vi "Test Refresh Active Path is First.vi"(8 "error in (no error)":errorcluster) -> (0 "error out":errorcluster)   [LabVIEW 2019]
uses:
  Setting Database/Setting Database.lvclass
  C:/Program Files (x86)/National Instruments/LabVIEW 2019/vi.lib/JKI/JKI SMO/SMO/SMO.lvclass
  ObjectSettings/ObjectSettings.lvclass/ObjectSettings.ctl
  ObjectSettings/Accessors/Read Enabled.vi
  ObjectSettings/Accessors/Write Enabled.vi
  Path Settings/Path Settings.lvclass
  C:/Users/Albro/Documents/GitHub/AFM-Lithography/lvsrc/Classes/Settings/ObjectSettings/ObjectSettings.lvclass
  <vilib>/addons/_JKI Toolkits/Caraya/classes/Assert/Assert Equal Value_Variant.vi
  <vilib>/addons/_JKI Toolkits/Caraya/classes/Test/Test.lvclass
  <vilib>/addons/_JKI Toolkits/Caraya/classes/Assert/Assert.lvclass
  <vilib>/JKI/JKI SMO/SMO/SMO.lvclass
  <vilib>/LabVIEW Open Source Project/Unicity/RandomStringGenerator/RandomStringGenerator.lvclass
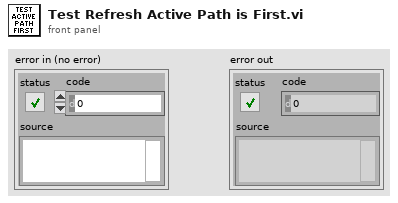
[diagram p1: front panel]
types:
  T1 = typedef "Setting Database.lvclass/PublicEvents--Cluster.ctl" = cluster{"NewActivePath":refnum<user-event>, "PathsUpdated":refnum<user-event>, "RectanglesUpdated":refnum<user-event>, "NewActiveRectangle":refnum<user-event>, "NewActiveFunnel":refnum<user-event>, "FunnelsUpdated":refnum<user-event>, "NewActiveDot":refnum<user-event>, "DotsUpdated":refnum<user-event>}
  T2 = typedef "Setting Database.lvclass/PrivateEvents--Setting Database.Refresh.ctl" = cluster{"Paths":string[], "Rectangles":string[], "Funnels":string[], "Dots":string[]}
  T3 = typedef "Setting Database.lvclass/PublicEvents--Setting Database.NewActivePath.ctl" = refnum<class "Path Settings.lvclass">
  T4 = typedef "Setting Database.lvclass/PublicEvents--Setting Database.PathsUpdated.ctl" = refnum<class "Path Settings.lvclass">[]
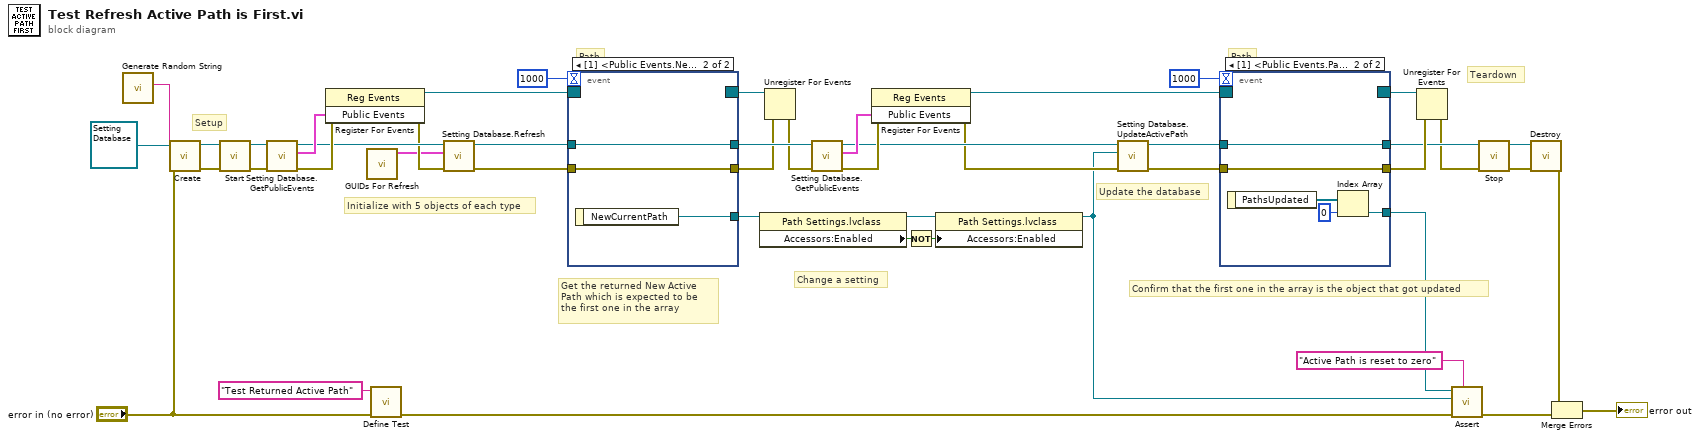
[diagram p0: block diagram]
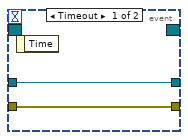
[diagram p2: hidden frame]
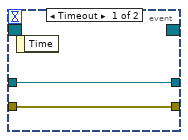
[diagram p3: hidden frame]
diagram:
  # "Confirm that the first one in the array is the object that got updated"
  # "Update the database"
  # "Change a setting"
  # "Get the returned New Active Path which is expected to be the first one in the array"
  # "Initialize with 5 objects of each type"
  # "Path"
  # "Path"
  # "Teardown"
  # "Setup"
  n1 = call <vilib>:"Generate Random String.vi"() -> ("Random String"=w1:string)  [unwired: 11 in]
  n2 = call <vilib>:"Create.vi"("error in (no error)"="error in (no error)", "Subsystem Name (optional)"=w1, "SMO"=refnum<class "Setting Database.lvclass"> refnum ("Setting Database.lvclass")) -> ("error out"=w43:errorcluster, "SMO out"=w36:refnum<class "Setting Database.lvclass">)  [unwired: 6 in, 1 out]
  n3 = call <vilib>:"Start.vi"("error in (no error)"=w43, "SMO"=w36) -> ("error out"=w42:errorcluster, "SMO out"=w35:refnum<class "Setting Database.lvclass">)  [unwired: 8 in]
  n4 = call "Setting Database.GetPublicEvents.vi"("error in (no error)"=w42, "Setting Database"=w35) -> ("error out"=w40:errorcluster, "Public Events"=w31:T1, "Setting Database out"=w28:refnum<class "Setting Database.lvclass">)  [unwired: 7 in]
  n5 = register-events(error in=w40, w31) -> (reference out=w29:refnum<event-registration>, error out=w26:errorcluster)  [unwired: 1 in]
  n6 = call "GUIDs For Refresh.vi"() -> ("Initialize"=w2:T2)  [unwired: 11 in]
  n7 = call <vilib>:"Define Test.vi"("error in (no error)"="error in (no error)", "Label (VI Title)"="Test Returned Active Path") -> ("error out"=w45:errorcluster)  [unwired: 8 in, 1 out]
  n8 = call "Setting Database.Refresh.vi"("error in (no error)"=w26, "Initialize"=w2, "Setting Database"=w28) -> ("error out"=w25:errorcluster, "Setting Database out"=w27:refnum<class "Setting Database.lvclass">)  [unwired: 7 in]
  n9 = event shown="[1] <Public Events.NewActivePath>: User Event" {
    selector: w29 -> [_ _]
    dyn-events: [_ _] -> w33
    timeout: 1000 -> [_ _]
    tunnel: [w48 w51] -> w23
    tunnel: w25 -> [w48 w51]
    tunnel: w27 -> [w47 w50]
    tunnel: [w47 w50] -> w24
    tunnel: [_ w49] -> w9
    event Timeout {
      n10 = event-data() -> ()  [unwired: 1 in, 1 out]
    }
    event User Event {
      n11 = event-data() -> ("NewCurrentPath"=w49:T3)  [unwired: 1 in]
    }
  }
  n12 = property on="Property Node" class="Path Settings.lvclass"(reference=w9) -> (reference out=w8:T3, "Accessors:Enabled"=w7:bool)  [unwired: 1 in, 1 out]
  n13 = Unregister For Events(event registration refnum=w33, error in=w23) -> (error out=w22:errorcluster)
  n14 = call "Setting Database.GetPublicEvents.vi"("error in (no error)"=w22, "Setting Database"=w24) -> ("error out"=w20:errorcluster, "Public Events"=w21:T1, "Setting Database out"=w13:refnum<class "Setting Database.lvclass">)  [unwired: 7 in]
  n15 = register-events(error in=w20, w21) -> (reference out=w16:refnum<event-registration>, error out=w11:errorcluster)  [unwired: 1 in]
  n16 = Not(x=w7) -> (.not. x?=w6:bool)
  n17 = property on="Property Node" class="Path Settings.lvclass"(reference=w8, "Accessors:Enabled"=w6) -> (reference out=w4:T3)  [unwired: 1 in, 1 out]
  n18 = call "Setting Database.UpdateActivePath.vi"("error in (no error)"=w11, "UpdateCurrentPath"=w4, "Setting Database"=w13) -> ("error out"=w10:errorcluster, "Setting Database"=w12:refnum<class "Setting Database.lvclass">)  [unwired: 7 in]
  n19 = event shown="[1] <Public Events.PathsUpdated>: User Event" {
    selector: w16 -> [_ _]
    dyn-events: [_ _] -> w17
    timeout: 1000 -> [_ _]
    tunnel: [w53 w58] -> w19
    tunnel: w10 -> [w53 w58]
    tunnel: w12 -> [w52 w57]
    tunnel: [w52 w57] -> w15
    tunnel: [_ w55] -> w5
    event Timeout {
      n20 = event-data() -> ()  [unwired: 1 in, 1 out]
    }
    event User Event {
      n21 = event-data() -> ("PathsUpdated"=w56:T4)  [unwired: 1 in]
      n22 = Index Array(array=w56, index=0) -> (element=w55:refnum<class "Path Settings.lvclass">)
    }
  }
  n23 = Unregister For Events(event registration refnum=w17, error in=w19) -> (error out=w14:errorcluster)
  n24 = call-poly <vilib>:"Assert.vi"("Label"="Active Path is reset to zero", "error in (no error)"=w45, "Actual"=w4, "Expected"=w5) -> ("error out"=w46:errorcluster)  [unwired: 6 in, 1 out]
  n25 = call <vilib>:"Stop.vi"("error in (no error)"=w14, "SMO"=w15) -> ("error out"=w41:errorcluster, "SMO out"=w34:refnum<class "Setting Database.lvclass">)  [unwired: 8 in]
  n26 = call <vilib>:"Destroy.vi"("error in (no error)"=w41, "SMO"=w34) -> ("error out"=w39:errorcluster)  [unwired: 9 in]
  n27 = Merge Errors(w39, w46) -> (→"error out":errorcluster)
